vi "Set References.vi"(4 "Car Position Simulation Ref":refnum<vi>, 6 "Active Option Ref":refnum<vi>, 11 "Car Position Simulation View Definition in":refnum<class "Car Position Simulation View Definition.lvclass">) -> (3 "Car Position Simulation View Definition out":refnum<class "Car Position Simulation View Definition.lvclass">)   [LabVIEW 2019, in "Car Position Simulation View Definition.lvclass"]
uses:
  <vilib>/gpm_packages/@cs/Car-wash/Source/Car Position Simulation View Definition/Car Position Simulation View Definition/Car Position Simulation View Definition.lvclass
  <vilib>/gpm_packages/@cs/Car-wash/Source/Car Position Simulation View Definition/Car Position Simulation View Definition/Car Position Simulation View Definition.lvclass/Car Position Simulation View Definition.ctl
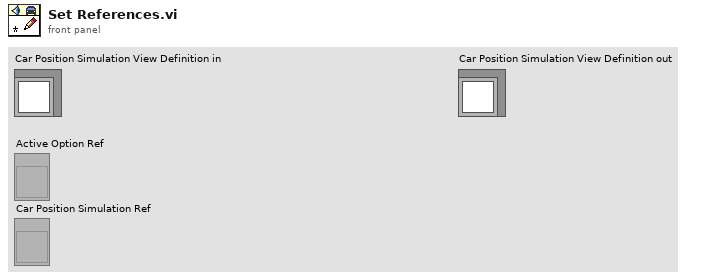
[diagram p1: front panel]
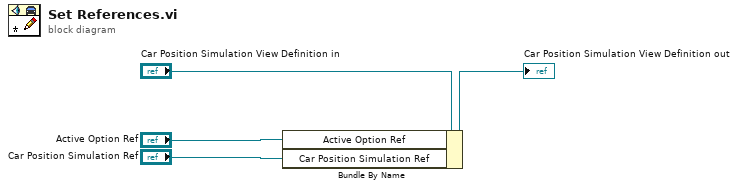
[diagram p0: block diagram]
diagram:
  n1 = Bundle By Name(cluster="Car Position Simulation View Definition in", "Active Option Ref"="Active Option Ref", "Car Position Simulation Ref"="Car Position Simulation Ref") -> (→"Car Position Simulation View Definition out":refnum<class "Car Position Simulation View Definition.lvclass">)
